vi "Set Acquisition Callback.vi"(8 "error in (no error)":errorcluster, 10 "vi reference":refnum<vi>, 11 "Camera_Prime95B in":refnum<class "Camera_Prime95B.lvclass">) -> (0 "error out":errorcluster, 3 "Camera_Prime95B out":refnum<class "Camera_Prime95B.lvclass">)   [LabVIEW 2020, in "Camera_Prime95B.lvlib" / "Camera_Prime95B.lvclass"]
uses:
  Camera_Prime95B.lvclass
  Camera_Prime95B.lvclass/Camera_Prime95B.ctl
  E:/Development/DevHardSoftware/MMicroscopyAF/Model/Real Hardware/Camera_Prime95B/Camera_Prime95B/Dependencies/PVCamNET.dll
  Dependencies/PVCamNET.dll
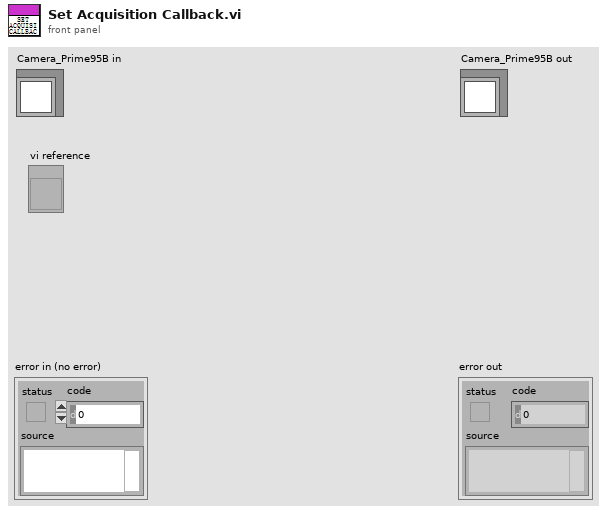
[diagram p1: front panel]
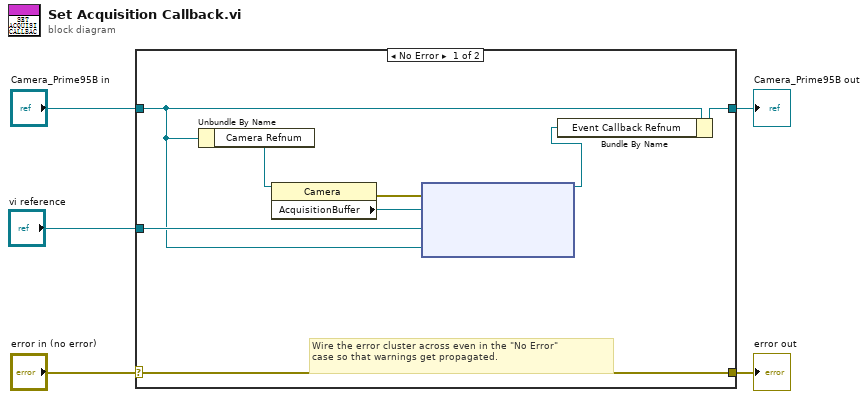
[diagram p0: block diagram]
diagram:
  n1 = case shown="No Error" "error in (no error)" {
    selector: "error in (no error)" -> [w13 w15]
    tunnel: [w13 w15] -> w4
    tunnel: [w7 w14] -> w2
    tunnel: "Camera_Prime95B in" -> [w9 w14]
    tunnel: "vi reference" -> [w10 _]
    frame No Error {
      # "Wire the error cluster across even in the \"No Error\"\ncase so that warnings get propagated."
      n2 = Unbundle By Name(w9) -> ("Camera Refnum"=w8:refnum<k24>)
      n3 = property class="Camera"(reference=w8) -> (error out=w12:errorcluster, "AcquisitionBuffer"=w11:refnum<k24>)  [unwired: 1 in, 1 out]
      n4 = node(w12, w11, w10, w9) -> (w6:refnum<k27>)  [unwired: 1 in, 1 out]
      n5 = Bundle By Name(cluster=w9, "Event Callback Refnum"=w6) -> (w7:refnum<class "Camera_Prime95B.lvclass">)
    }
    frame Error {
    }
  }
  "error out" <- w4
  "Camera_Prime95B out" <- w2
